vi "MockDigitalInput.vi"(11 "MockDigitalInput":T1={"BufferUpdateFIFO"="MockDigitalInputCommand"}) -> ()   [LabVIEW 2016, in "FPGAMockDigitalInput.lvlib"]
uses:
  FPGAMockDigitalInput.lvlib
  DataTypes/MockDigitalInputSettings.ctl
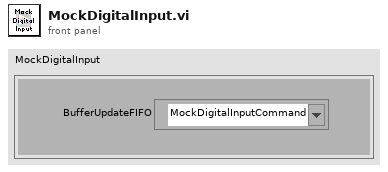
[diagram p1: front panel]
types:
  T1 = typedef "FPGAMockDigitalInput.lvlib/MockDigitalInputSettings.ctl" = cluster{"BufferUpdateFIFO":refnum<k21>}
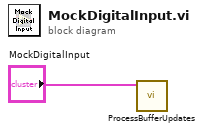
[diagram p0: block diagram]
diagram:
  n1 = call "ProcessBufferUpdates.vi"("MockDigitalInput"="MockDigitalInput") -> ()  [unwired: 11 in]
